vi "Measure IV curves.vi"() -> ()   [LabVIEW 2014]
uses:
  Environmental Chamber LabVIEW and Instruments/Drivers and Software/LabVIEW 8.2 Drivers/keithley_24xx/Keithley 24XX/Public/Data/Read (Single Point).vi
  <vilib>/Utility/file.llb/Write To Spreadsheet File (string).vi
  Environmental Chamber LabVIEW and Instruments/Drivers and Software/keithley_24xx/Keithley 24XX/Keithley 24XX.lvlib
panel:
  in  "voltage settings":T1={"Vi (V)"=0.0, "Vf (V)"=0.3, "steps"=30.0, "Number of curves"=1, "Delay (min)"=0.05} {"Delay (min)" min=0.0 format="%#_13g"; "Number of curves" step=1}
  out "File path":path
  in  "STOP":bool
  out "V":dbl
  out "2420 IV curve":cluster{"X":dbl[], "Y":dbl[]}[](graph)
  out "I":sgl
  out "R":sgl
  in  "File notes":string
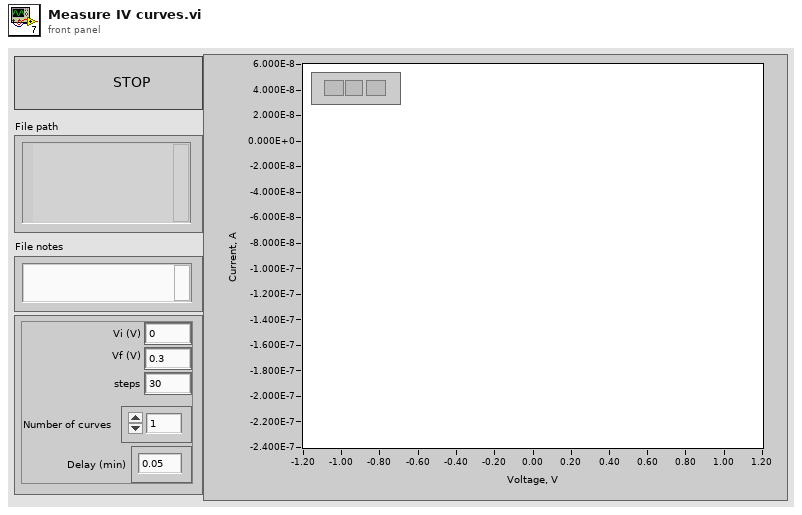
[diagram p1: front panel]
types:
  T1 = cluster{"Vi (V)":dbl, "Vf (V)":dbl, "steps":dbl, "Number of curves":u32, "Delay (min)":dbl}
  T2 = enum16{"open", "replace", "create", "open or create", "replace or create", "replace or create with confirmation"}
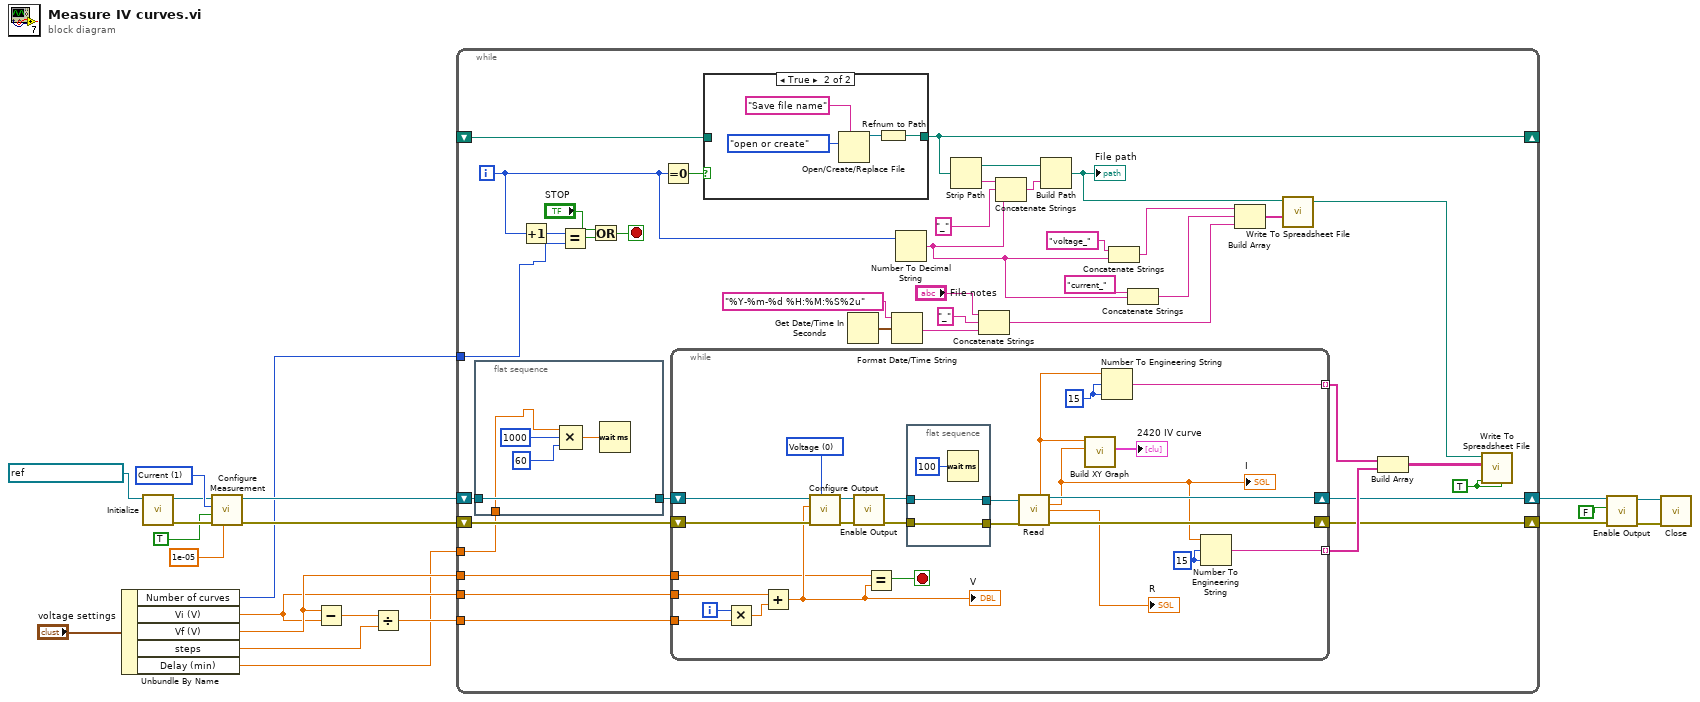
[diagram p0: block diagram]
diagram:
  w13 = u16 1 items=["Volts", "Current", "Resistance"] ("Function (0: Volts)")
  n1 = Unbundle By Name("voltage settings") -> ("Number of curves"=w2:u32, "Vi (V)"=w3:dbl, "Vf (V)"=w4:dbl, "steps"=w5:dbl, "Delay (min)"=w1:dbl)
  n2 = call "Initialize.vi"("VISA resource name"=refnum<visa-resource-name> "GPIB1::24::INSTR") -> ("error out"=w9:errorcluster, "VISA resource name out"=w10:refnum<visa-resource-name>)  [unwired: 9 in]
  n3 = call "Configure Measurement.vi"("Manual Range (1.0)"=1e-05, "error in (no error)"=w9, "Enable Auto Range (T:Enable)"=TRUE, "Function (0: Volts)"=w13, "VISA resource name"=w10) -> ("error out"=w12:errorcluster, "VISA resource name out"=w11:refnum<visa-resource-name>)  [unwired: 5 in]
  n4 = Subtract(x=w4, y=w3) -> (x-y=w21:dbl)
  n5 = Divide(x=w21, y=w5) -> (x/y=w20:dbl)
  n6 = while {
    tunnel: w4 -> [w61]
    tunnel: w3 -> [w60]
    tunnel: w20 -> [w59]
    shift-right: [w51] -> w15
    shift-left: w12 -> [w50]
    shift-right: [w52] -> w16
    shift-left: w11 -> [w31]
    shift-right: [w40] -> _
    shift-left: _ -> [w41]
    tunnel: w2 -> [w23]
    tunnel: w1 -> [w22]
    i -> [w43]
    stop <- w47 stop-if-true
    w58 = TRUE ("transpose? (no:F)")
    n7 = flat-sequence {
      tunnel: [w66] -> w30
      tunnel: w31 -> [w66]
      tunnel: w22 -> [w62]
      frame #0 {
        n8 = Compound Arithmetic op=MULTIPLY(w62, u32 1000 ("value"), u32 60 ("value")) -> (w65:dbl)
        n9 = Wait (ms)(milliseconds to wait=w65) -> ()  [unwired: 1 out]
      }
    }
    n10 = Increment(x=w43) -> (x+1=w45:i32)
    n11 = Equal?(x=w45, y=w23) -> (x = y?=w44:bool)
    n12 = Or(x="STOP", y=w44) -> (x .or. y?=w47:bool)
    n13 = Equal To 0?(x=w43) -> (x = 0?=w42:bool)
    n14 = while {
      tunnel: [w90] -> w54 mode=indexing
      shift-right: [w96] -> w51
      shift-left: w50 -> [w95]
      shift-right: [w97] -> w52
      shift-left: w30 -> [w94]
      tunnel: w59 -> [w72]
      tunnel: w60 -> [w85]
      tunnel: [w84] -> w55 mode=indexing
      tunnel: w61 -> [w74]
      i -> [w73]
      stop <- w76 stop-if-true
      w80 = i16 15 ("precision (6)")
      w81 = i16 15 ("precision (6)")
      w91 = u16 0 items=["Voltage", "Current"] ("Source Mode  (0: Voltage)")
      n15 = Multiply(x=w73, y=w72) -> (x*y=w83:dbl)
      n16 = Add(x=w85, y=w83) -> (x+y=w75:dbl)
      "V" <- w75
      n17 = call "Configure Output.vi"("Source Mode  (0: Voltage)"=w91, "error in (no error)"=w95, "Output Level (0)"=w75, "VISA resource name"=w94) -> ("error out"=w93:errorcluster, "VISA resource name out"=w92:refnum<visa-resource-name>)  [unwired: 6 in]
      n18 = call "Enable Output.vi"("error in (no error)"=w93, "VISA resource name"=w92) -> ("error out"=w86:errorcluster, "VISA resource name out"=w89:refnum<visa-resource-name>)  [unwired: 8 in]
      n19 = Equal?(x=w74, y=w75) -> (x = y?=w76:bool)
      n20 = flat-sequence {
        tunnel: [w100] -> w88
        tunnel: w89 -> [w100]
        tunnel: w86 -> [w99]
        tunnel: [w99] -> w87
        frame #0 {
          n21 = Wait (ms)(milliseconds to wait=u32 100) -> ()  [unwired: 1 out]
        }
      }
      n22 = call-poly "Read.vi"("VISA resource name"=w88, "error in (no error)"=w87) -> ("Voltage"=w78:sgl, "VISA resource name out"=w97:refnum<visa-resource-name>, "Current"=w79:sgl, "Resistance"=→"R":sgl, "error out"=w96:errorcluster)  [unwired: 7 in, 2 out]
      "I" <- w79
      n23 = call "Build XY Graph"("Y Input"=w79, "X Input"=w78) -> ("XY Graph"=→"2420 IV curve":cluster{"X":dbl[], "Y":dbl[]}[])  [unwired: 8 in, 1 out]
      n24 = Number To Engineering String(2:w80, 3:w80, 4:w78) -> (0:w84:string)  [unwired: 1 in]
      n25 = Number To Engineering String(2:w81, 3:w81, 4:w79) -> (0:w90:string)  [unwired: 1 in]
    }
    n26 = case shown="True" w42 {
      tunnel: [w67 w68] -> w40
      tunnel: w41 -> [w67 _]
      frame False {
      }
      frame True {
        n27 = Open/Create/Replace File(prompt="Save file name", operation (0:open)=T2."open or create") -> (refnum out=w69:refnum<file>)  [unwired: 4 in, 2 out]
        n28 = Refnum to Path(1:w69) -> (0:w68:path)
      }
    }
    n29 = Get Date/Time In Seconds() -> (seconds since 1Jan1904=w36:timestamp)
    n30 = Format Date/Time String(time format string (%c)="%Y-%m-%d %H:%M:%S%2u", seconds (now)=w36) -> (date/time string=w32:string)  [unwired: 1 in]
    n31 = Number To Decimal String(number=w43) -> (decimal integer string=w26:string)  [unwired: 1 in]
    n32 = Strip Path(path=w40) -> (stripped path=w39:path, name=w38:string)
    n33 = Concatenate Strings("File notes", "_" ("string"), w32) -> (w33:string)
    n34 = Concatenate Strings(w38, "_" ("string"), w26) -> (w29:string)
    n35 = Build Path(base path=w39, name or relative path=w29) -> (appended path=w49:path)
    "File path" <- w49
    n36 = Concatenate Strings("voltage_", w26) -> (w24:string)
    n37 = Concatenate Strings("current_", w26) -> (w27:string)
    n38 = Build Array(w24, w27, w33) -> (w57:string[])
    n39 = call-poly <vilib>:"Write To Spreadsheet File.vi"("1D data"=w57, "file path (dialog if empty)"=w49) -> ("new file path (Not A Path if cancelled)"=w56:path)  [unwired: 6 in]
    n40 = Build Array(w55, w54) -> (w53:string[][])
    n41 = call-poly <vilib>:"Write To Spreadsheet File.vi"("transpose? (no:F)"=w58, "append to file? (new file:F)"=w58, "2D data"=w53, "file path (dialog if empty)"=w56) -> ()  [unwired: 4 in, 1 out]
  }
  n42 = call "Enable Output.vi"("error in (no error)"=w15, "Enable Output (T: Enable)"=FALSE, "VISA resource name"=w16) -> ("error out"=w17:errorcluster, "VISA resource name out"=w19:refnum<visa-resource-name>)  [unwired: 7 in]
  n43 = call "Close.vi"("error in (no error)"=w17, "VISA resource name"=w19) -> ()  [unwired: 9 in, 1 out]
